vi "IntakeExecuteLogic.vi"(9 "HaveAlgaeSensor":bool, 11 "HaveCoralSensor":bool) -> (1 "MotorDemandRight":dbl, 2 "MotorDemandLeft":dbl, 3 "MotorDemandTop":dbl, 4 "CurrentState":T1)   [LabVIEW 2023]
doc: "Intake Commands go in and Motor Demands are outputted\nOutputs:\n--MotorDemandTop--numeric\n--MotorDemandLeft--numeric\nMotorDemandRight--numeric"
uses:
  IntakeStates.ctl
  <vilib>/Rock Robotics/WPI/ThirdParty/JAS_Junk/TrajLib/VI/BoolCmd_Recv_Internal.vi
  <vilib>/Rock Robotics/WPI/ThirdParty/JAS_Junk/TrajLib/VI/DigSeqLogic_Edge_On.vi
  <vilib>/Rock Robotics/WPI/ThirdParty/JAS_Junk/TrajLib/VI/BoolCmd_ObtainQueue.vi
  IntakeGlobal.vi
  <vilib>/Rock Robotics/WPI/ThirdParty/JAS_Junk/TrajLib/Trajectory_Library.lvlib
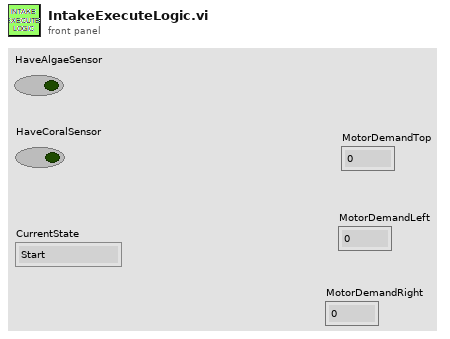
[diagram p1: front panel]
types:
  T1 = typedef "IntakeStates.ctl" = enum16{"Start", "WaitForCommand", "IntakeCoral", "IntakeAlgae", "WaitForCoral", "WaitForAlgae", "DepositCoral", "DepositAlgae", "DepositCoralTimer", "DepositAlgaeTimer"}
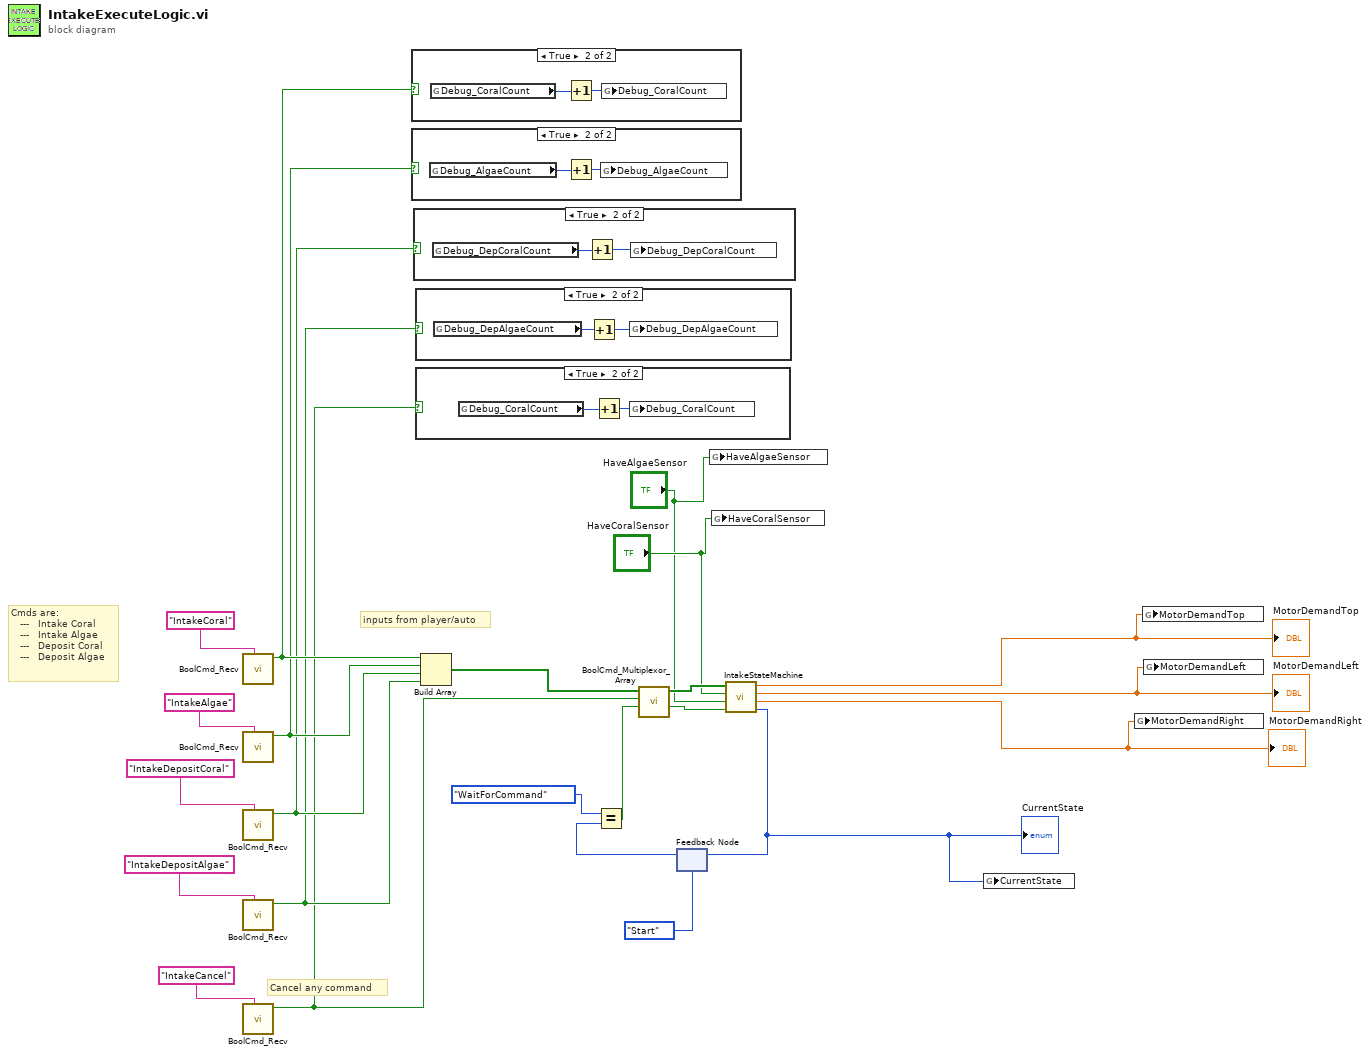
[diagram p0: block diagram]
diagram:
  # "Cmds are:\n   ---   Intake Coral\n   ---   Intake Algae\n   ---   Deposit Coral\n   ---   Deposit Algae"
  # "inputs from player/auto"
  # "Cancel any command"
  n1 = call <vilib>:"BoolCmd_Recv.vi"("Command Name"="IntakeCoral") -> ("New Request"=w5:bool)  [unwired: 9 in, 1 out]
  n2 = call <vilib>:"BoolCmd_Recv.vi"("Command Name"="IntakeAlgae") -> ("New Request"=w4:bool)  [unwired: 9 in, 1 out]
  n3 = call <vilib>:"BoolCmd_Recv.vi"("Command Name"="IntakeDepositCoral") -> ("New Request"=w3:bool)  [unwired: 9 in, 1 out]
  n4 = call <vilib>:"BoolCmd_Recv.vi"("Command Name"="IntakeDepositAlgae") -> ("New Request"=w2:bool)  [unwired: 9 in, 1 out]
  n5 = call <vilib>:"BoolCmd_Recv.vi"("Command Name"="IntakeCancel") -> ("New Request"=w1:bool)  [unwired: 9 in, 1 out]
  n6 = case shown="True" w5 {
    frame False {
    }
    frame True {
      n7 = global read "IntakeGlobal.vi" "Debug_CoralCount"() -> (w25:i32)
      n8 = Increment(x=w25) -> (x+1=w24:i32)
      n9 = global write "IntakeGlobal.vi" "Debug_CoralCount"(w24) -> ()
    }
  }
  n10 = case shown="True" w4 {
    frame False {
    }
    frame True {
      n11 = global read "IntakeGlobal.vi" "Debug_AlgaeCount"() -> (w27:i32)
      n12 = Increment(x=w27) -> (x+1=w26:i32)
      n13 = global write "IntakeGlobal.vi" "Debug_AlgaeCount"(w26) -> ()
    }
  }
  n14 = case shown="True" w3 {
    frame False {
    }
    frame True {
      n15 = global read "IntakeGlobal.vi" "Debug_DepCoralCount"() -> (w29:i32)
      n16 = Increment(x=w29) -> (x+1=w28:i32)
      n17 = global write "IntakeGlobal.vi" "Debug_DepCoralCount"(w28) -> ()
    }
  }
  n18 = case shown="True" w2 {
    frame False {
    }
    frame True {
      n19 = global read "IntakeGlobal.vi" "Debug_DepAlgaeCount"() -> (w31:i32)
      n20 = Increment(x=w31) -> (x+1=w30:i32)
      n21 = global write "IntakeGlobal.vi" "Debug_DepAlgaeCount"(w30) -> ()
    }
  }
  n22 = case shown="True" w1 {
    frame False {
    }
    frame True {
      n23 = global read "IntakeGlobal.vi" "Debug_CoralCount"() -> (w33:i32)
      n24 = Increment(x=w33) -> (x+1=w32:i32)
      n25 = global write "IntakeGlobal.vi" "Debug_CoralCount"(w32) -> ()
    }
  }
  n26 = Build Array(w5, w4, w3, w2) -> (w20:bool[])
  n27 = feedback #1(IntakeStates."Start" ("CurrentState")) -> (w15:T1)
  n28 = Equal?(x=IntakeStates."WaitForCommand", y=w15) -> (x = y?=w13:bool)
  n29 = call <vilib>:"BoolCmd_Multiplexor_Array.vi"("Ready"=w13, "Command Cancel"=w1, "Commands"=w20) -> ("Do Cancel"=w17:bool, "Do Command"=w18:bool[])  [unwired: 7 in]
  n30 = global write "IntakeGlobal.vi" "HaveAlgaeSensor"("HaveAlgaeSensor") -> ()
  n31 = global write "IntakeGlobal.vi" "HaveCoralSensor"("HaveCoralSensor") -> ()
  n32 = call "IntakeStateMachine.vi"("IntakeCancel"=w17, "HaveAlgaeSensor"="HaveAlgaeSensor", "HaveCoralSensor"="HaveCoralSensor", "IntakeCommands"=w18) -> ("CurrentState"=w6:T1, "RightMotorDemand"=w9:dbl, "LeftMotorDemand"=w10:dbl, "TopMotorDemand"=w11:dbl)  [unwired: 4 in]
  "MotorDemandLeft" <- w10
  "MotorDemandRight" <- w9
  "CurrentState" <- w6
  "MotorDemandTop" <- w11
  n33 = feedback-in #1(w6) -> ()
  n34 = global write "IntakeGlobal.vi" "CurrentState"(w6) -> ()
  n35 = global write "IntakeGlobal.vi" "MotorDemandRight"(w9) -> ()
  n36 = global write "IntakeGlobal.vi" "MotorDemandTop"(w11) -> ()
  n37 = global write "IntakeGlobal.vi" "MotorDemandLeft"(w10) -> ()
